vi "Log msTick Timer.vi"(8 "error in (no error)":errorcluster, 11 "DbgTimers in":refnum<class "DbgTimers.lvclass">) -> (0 "error out":errorcluster, 2 "last Q entry":string, 3 "DbgTimers out":refnum<class "DbgTimers.lvclass">)   [LabVIEW 2017, in "DbgTimers.lvclass"]
doc: "Developed by Kevin Thompson\nkevin@thompsonengineering.net\n\nCopyright 2018-2020\nThompson Engineering, LLC"
uses:
  DbgTimers.lvclass
  DbgTimers.lvclass/DbgTimers.ctl
  Accessors/Get ObjData.vi
  <userlib>/_OpenG.lib/file/file.llb/File Exists - Scalar__ogtk.vi
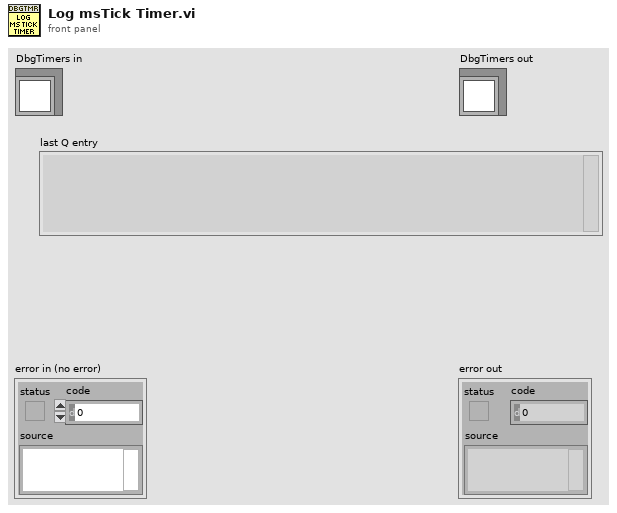
[diagram p1: front panel]
types:
  T1 = typedef "DbgTimers.lvclass/ObjData--cluster.ctl" = cluster{"Settings":T2, "ReadData-placeholder":T3, "Timers":T4, "Enable msTick Logging":bool, "LogFile_msTickTimer":path}
  T2 = typedef "DbgTimers.lvclass/Settings--cluster.ctl" = cluster{"Simulation":bool, "DbgTimer LogFolder":path}
  T3 = typedef "DbgTimers.lvclass/Read Data--cluster.ctl" = cluster{"Data":dbl}
  T4 = typedef "DbgTimers.lvclass/Timers--cluster.ctl" = cluster{"ms tick timers":T5[]}
  T5 = typedef "DbgTimers.lvclass/Millisecond Tick Timer--cluster.ctl" = cluster{"startTick":u32, "currentTick":u32, "elapsedTicks":u32, "totalElapsedTicks":u32}
  T6 = typedef "DbgTimers.lvclass/Millsecond Tick Timer Qdata--cluster.ctl" = cluster{"Time Stamp":timestamp, "comment":string, "idx":i32, "ms tick timer":T5}
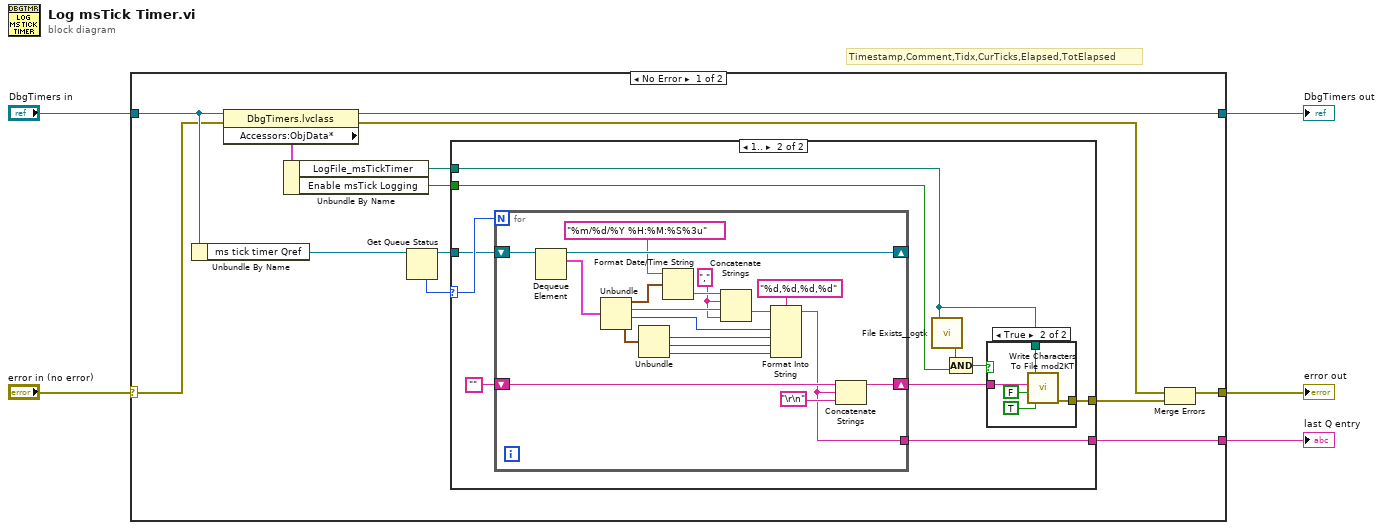
[diagram p0: block diagram]
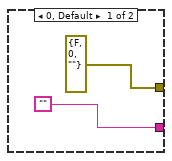
[diagram p2: hidden frame]
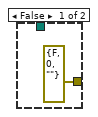
[diagram p3: hidden frame]
diagram:
  # "Timestamp,Comment,Tidx,CurTicks,Elapsed,TotElapsed"
  n1 = case shown="No Error" "error in (no error)" {
    selector: "error in (no error)" -> [w10 w57]
    tunnel: [w9 w57] -> w4
    tunnel: [w14 w56] -> w2
    tunnel: "DbgTimers in" -> [w18 w56]
    tunnel: [w11 _] -> w1
    frame No Error {
      n2 = Unbundle By Name(w18) -> ("ms tick timer Qref"=w17:refnum<queue>)
      n3 = property class="DbgTimers.lvclass"(reference=w18, error in=w10) -> (reference out=w14:refnum<class "DbgTimers.lvclass">, error out=w7:errorcluster, "Accessors:ObjData*"=w13:T1)
      n4 = Unbundle By Name(w13) -> ("LogFile_msTickTimer"=w12:path, "Enable msTick Logging"=w6:bool)
      n5 = Get Queue Status(queue=w17) -> (queue out=w15:refnum<queue>, # elements in queue=w16:i32)  [unwired: 2 in, 6 out]
      n6 = case shown="1.." w16 {
        selector: w16 -> [_ w30]
        tunnel: w15 -> [_ w29]
        tunnel: w12 -> [_ w21]
        tunnel: ["" w26] -> w11
        tunnel: [errorcluster {"status"=FALSE, "code"=0, "source"=""} ("error out") w25] -> w8
        tunnel: w6 -> [_ w23]
        frame 0, Default {
        }
        frame 1.. {
          n7 = for {
            N: w30 -> [_]
            shift-right: [w54] -> _
            shift-left: w29 -> [w55]
            shift-right: [w40] -> w27
            shift-left: "" -> [w39]
            tunnel: [w37] -> w26
            w42 = ","
            n8 = Dequeue Element(queue=w55) -> (queue out=w54:refnum<queue>, element=w53:T6)  [unwired: 2 in, 2 out]
            n9 = Unbundle(w53) -> ("Time Stamp"=w52:timestamp, "comment"=w49:string, "idx"=w47:i32, "ms tick timer"=w43:T5)
            n10 = Unbundle(w43) -> ("currentTick"=w46:u32, "elapsedTicks"=w45:u32, "totalElapsedTicks"=w44:u32)  [unwired: 1 out]
            n11 = Format Date/Time String(time format string (%c)="%m/%d/%Y %H:%M:%S%3u", seconds (now)=w52) -> (date/time string=w50:string)  [unwired: 1 in]
            n12 = Concatenate Strings(w50, w42, w49, w42) -> (w48:string)
            n13 = Format Into String(format string="%d,%d,%d,%d", initial string=w48, w47, w46, w45, w44) -> (resulting string=w37:string)  [unwired: 1 in, 1 out]
            n14 = Concatenate Strings(w39, w37, "\r\n") -> (w40:string)
          }
          n15 = call-poly <userlib>:"File Exists__ogtk.vi"("file path"=w21) -> ("exists"=w22:bool)  [unwired: 6 in, 1 out]
          n16 = Compound Arithmetic op=AND(w22, w23) -> (w24:bool)
          n17 = case shown="True" w24 {
            tunnel: w27 -> [_ w36]
            tunnel: w21 -> [_ w33]
            tunnel: [errorcluster {"status"=FALSE, "code"=0, "source"=""} ("error out") w32] -> w25
            frame False {
            }
            frame True {
              n18 = call <vilib>:"Write Characters To File mod2KT.vi"("append to file? (new file:F)"=TRUE, "advisory dialog? (display:T)"=FALSE, "character string"=w36, "file path (dialog if empty)"=w33) -> ("error out"=w32:errorcluster)  [unwired: 2 in, 1 out]
            }
          }
        }
      }
      n19 = Merge Errors(w7, w8) -> (w9:errorcluster)
    }
    frame Error {
    }
  }
  "error out" <- w4
  "DbgTimers out" <- w2
  "last Q entry" <- w1
